vi "New_probe_ver6-rev_with_cycle.vi"() -> ()   [LabVIEW 2012]
panel:
  in  "Period [ms]":dbl=100.0
  in  "wait for stable [ms]":dbl=100.0
  in  "I for Lockin [A]":dbl
  out "X-Y":cluster{"X":dbl[], "Y":dbl[]}[](graph) caption="XY Graph"
  out "R 2":cluster{"X":dbl[], "Y":dbl[]}[](graph) caption="XY Graph"
  out "Lockin Y (V)":dbl=0.0511149801
  out "H":cluster{"X":dbl[], "Y":dbl[]}[](graph) caption="XY Graph"
  in  "X":string(combo)="100 uA"
  out "Lakeshore Reading (K)":dbl
  in  "Measure":bool
  in  "Y":string(combo)="100 uA"
  out "T":cluster{"X":dbl[], "Y":dbl[]}[](graph) caption="XY Graph"
  in  "Reset":bool
  out "R":cluster{"X":dbl[], "Y":dbl[]}[](graph) caption="XY Graph"
  in  "T:Lock in\nF:delta":bool
  out "Lockin X (V)":dbl=0.0511149801
  in  "Lockin SR830":refnum<visa-resource-name>="GPIB0::22::INSTR"
  in  "Keithley":refnum<visa-resource-name>="GPIB0::20::INSTR"
  in  "Arm Delta":bool
  in  "I-HIGH [A]":dbl=0.0001 format="%#_6e"
  in  "DELAY [sec]":dbl=0.002 format="%#_6e"
  in  "Compliance [V]":dbl=1.0 format="%#_6f"
  in  "Abort Delta":bool
  out "Delta Reading [Ohm]":dbl=0.0511149801
  in  "Input (0: A  1: B)":u16
  in  "Stop":bool
  in  "Lakeshore":refnum<visa-resource-name>="GPIB0::12::INSTR"
  in  "ramp [mT/sec]":dbl=3.0
  in  "step [ms]":dbl=100.0
  in  "set [mT]":dbl
  in  "Set field":bool
  in  "Initialize":bool
  out "Magnetic Field [mT]":dbl(knob) scale=-500.0..500.0
  in  "Save":bool
  in  "?":bool
  in  "error in (no error)":errorcluster
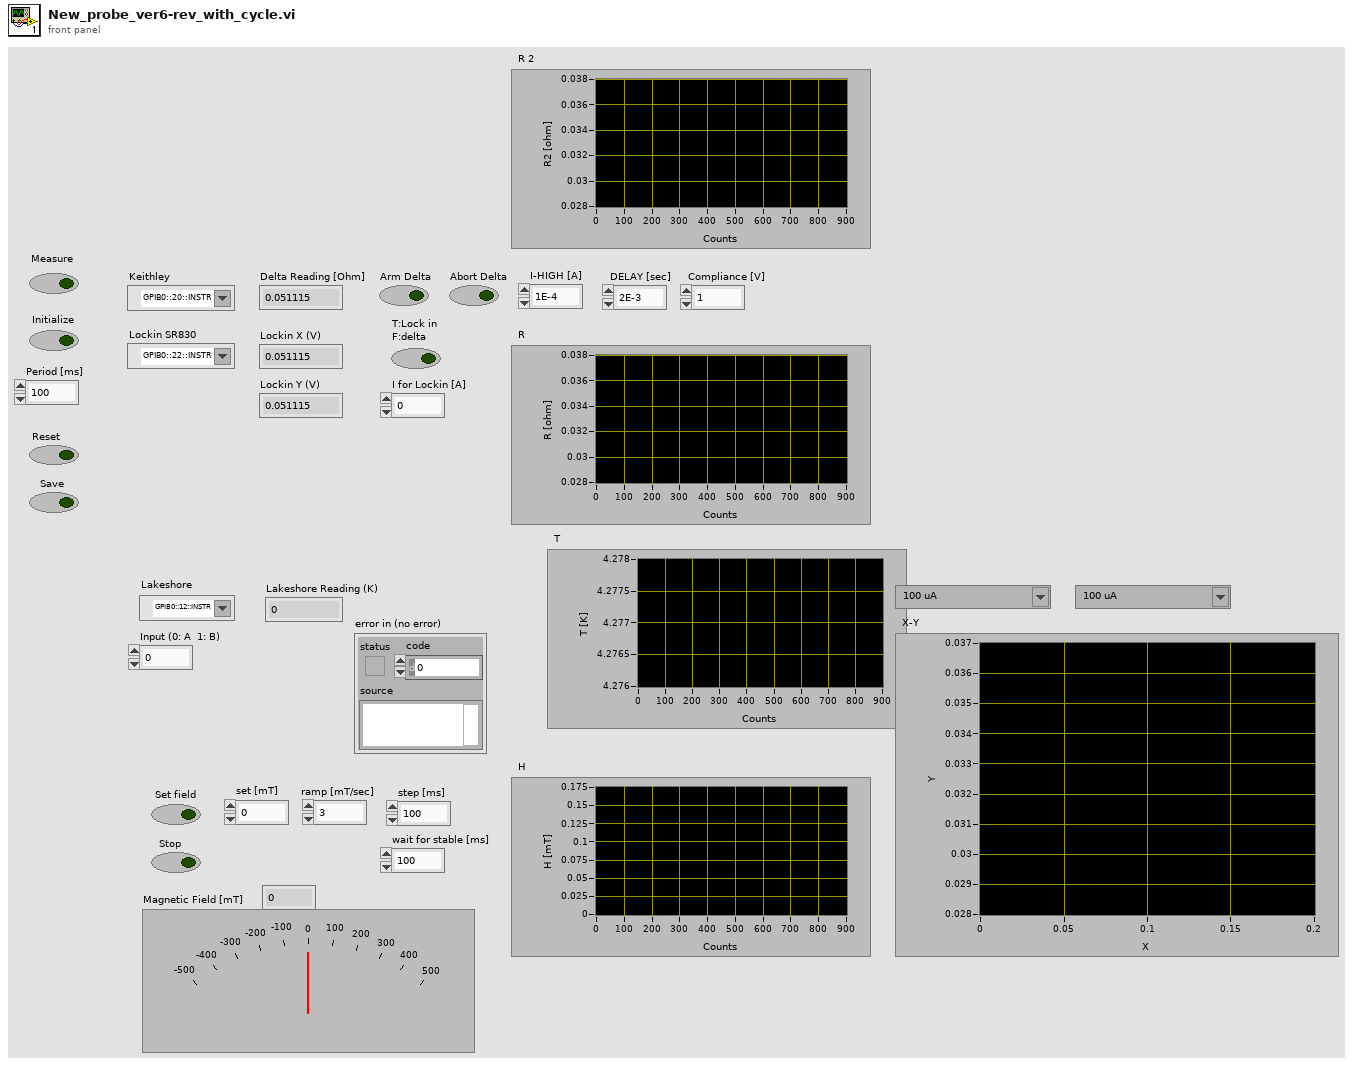
[diagram p1: front panel]
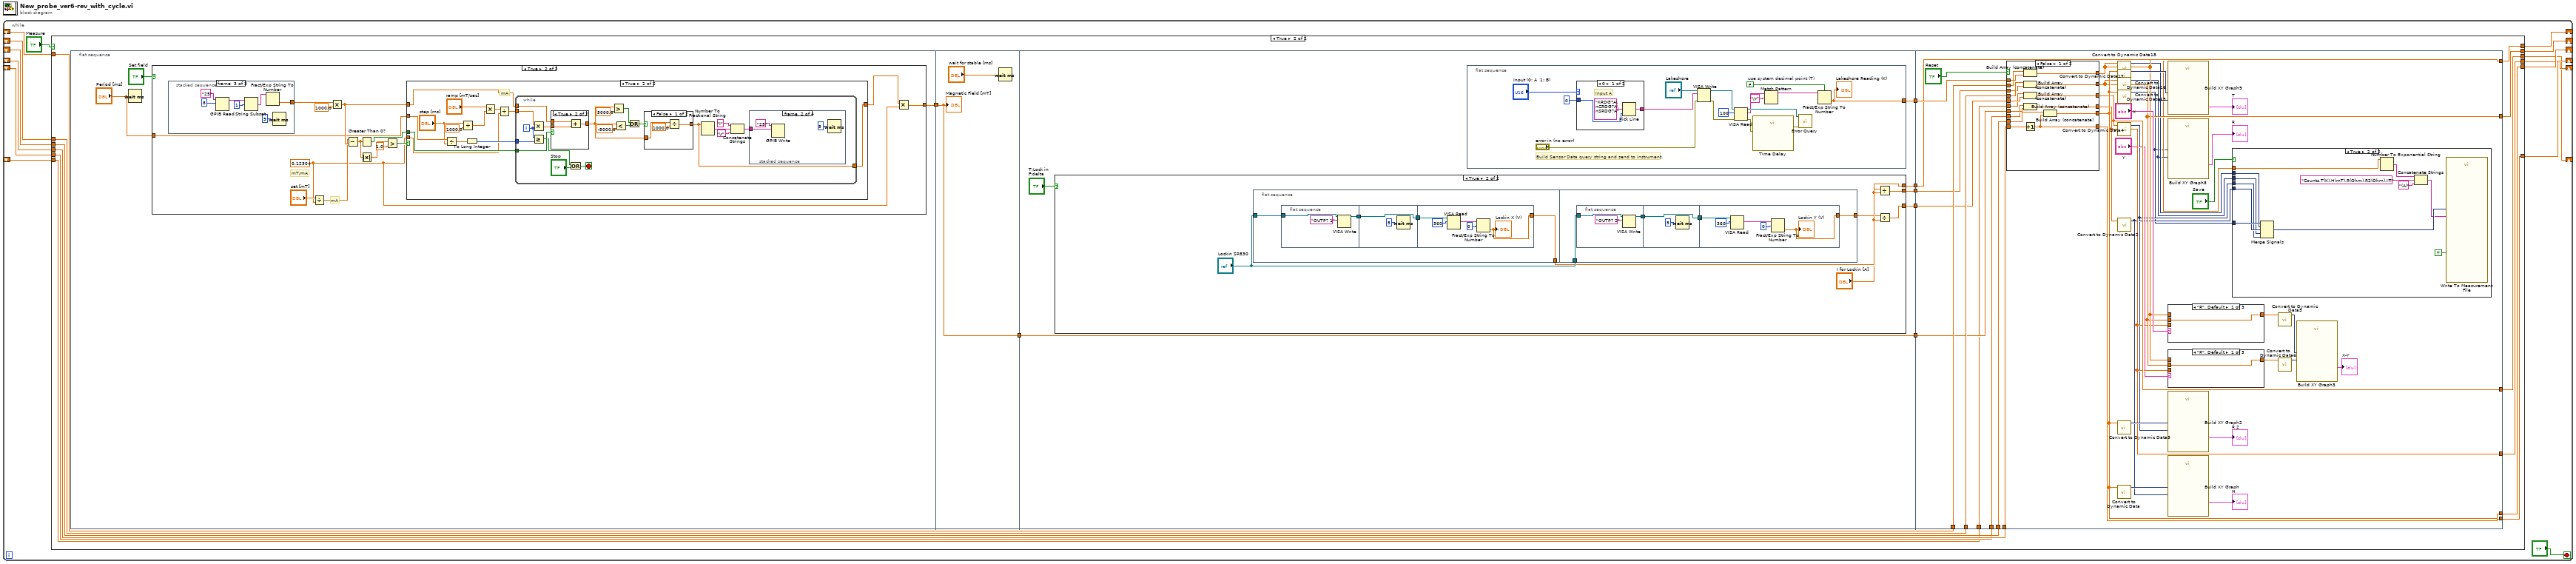
[diagram p0: block diagram]
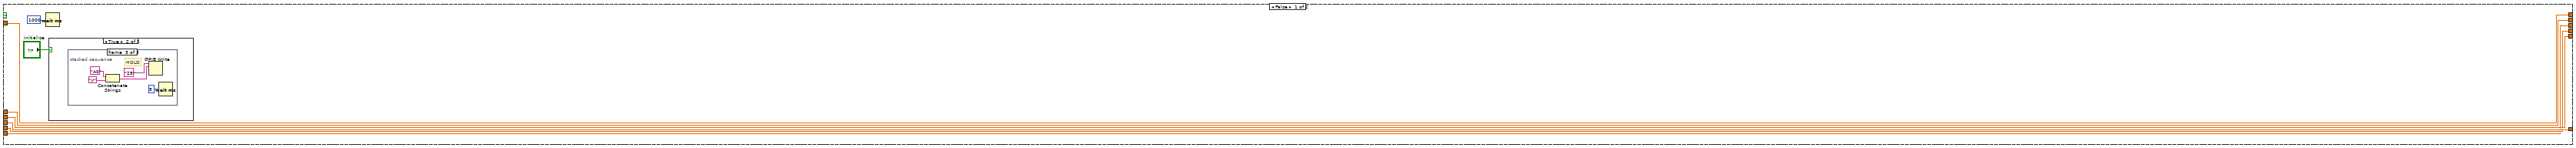
[diagram p2: hidden frame]
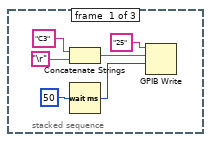
[diagram p4: hidden frame]
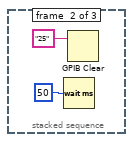
[diagram p5: hidden frame]
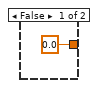
[diagram p6: hidden frame]
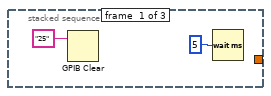
[diagram p7: hidden frame]
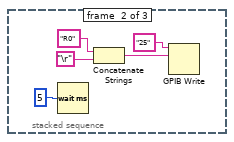
[diagram p8: hidden frame]
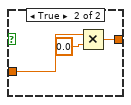
[diagram p10: hidden frame]
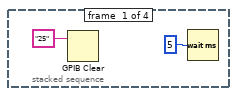
[diagram p11: hidden frame]
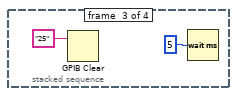
[diagram p12: hidden frame]
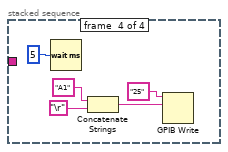
[diagram p13: hidden frame]
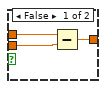
[diagram p14: hidden frame]
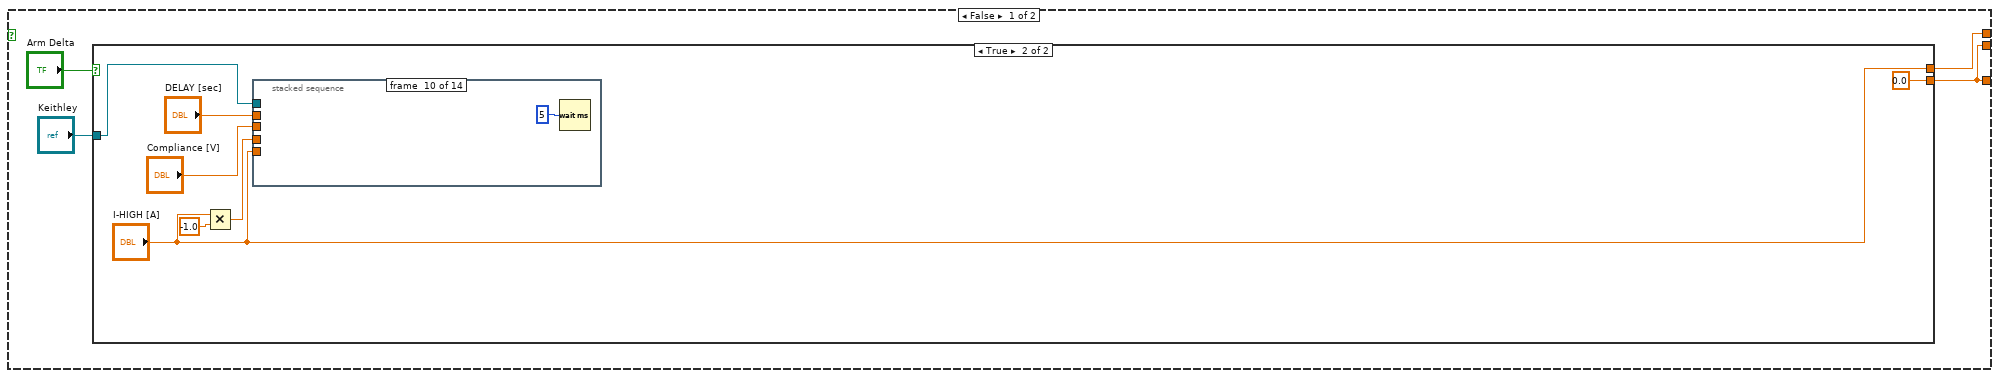
[diagram p15: hidden frame]
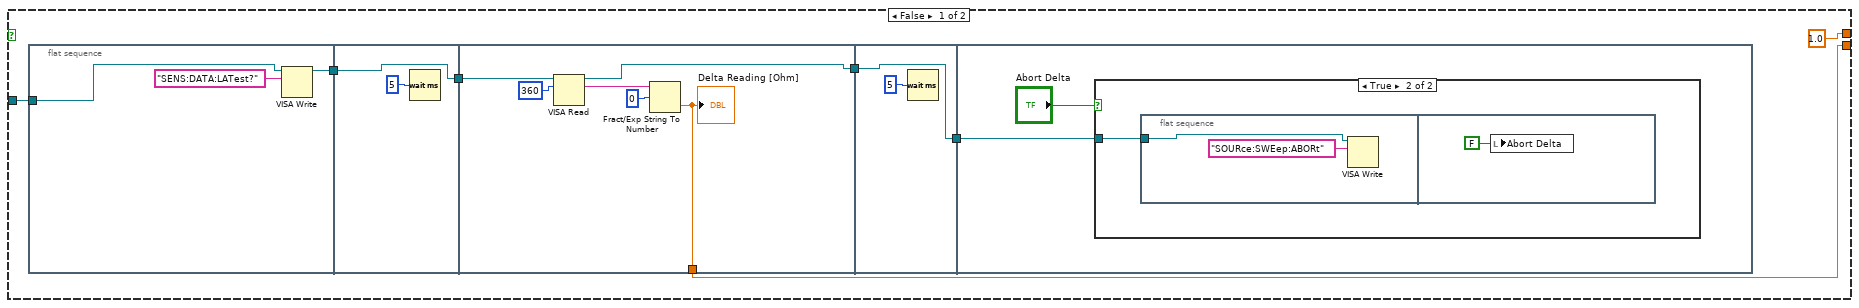
[diagram p16: hidden frame]
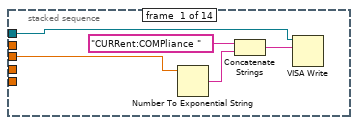
[diagram p18: hidden frame]
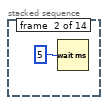
[diagram p19: hidden frame]
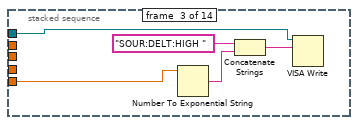
[diagram p20: hidden frame]
diagram:
  n1 = while {
    shift-right: [w13] -> _
    shift-left: _ -> [w6]
    shift-right: [w11] -> _
    shift-left: _ -> [w9]
    shift-right: [w10] -> _
    shift-left: _ -> [w8]
    shift-right: [w12] -> _
    shift-left: _ -> [w7]
    shift-right: [w4] -> _
    shift-left: _ -> [w3]
    shift-right: [w2] -> _
    shift-left: _ -> [w1]
    stop <- "?" stop-if-true
    n2 = case shown="True" "Measure" {
      tunnel: [w20 w51] -> w13
      tunnel: [w18 w50] -> w12
      tunnel: [w19 w49] -> w11
      tunnel: [w17 w48] -> w10
      tunnel: w9 -> [w19 w44]
      tunnel: w8 -> [w17 w45]
      tunnel: w7 -> [w18 w46]
      tunnel: w6 -> [w20 w47]
      tunnel: [w16 w41] -> w4
      tunnel: w3 -> [w16 w40]
      tunnel: [w15 w38] -> w2
      tunnel: w1 -> [w15 w37]
      frame False {
        n3 = Wait (ms)(milliseconds to wait=u32 1000) -> ()  [unwired: 1 out]
        n4 = case shown="True" "Initialize" {
          frame False {
          }
          frame True {
            n5 = stacked-sequence {
              frame #0 {
                n6 = Concatenate Strings("C3", "\r") -> (w24:string)
                n7 = Wait (ms)(milliseconds to wait=50) -> (millisecond timer value=w25:u32)
                n8 = GPIB Write(0:"25", 1:w24, 2:w25) -> ()  [unwired: 2 in, 2 out]
              }
              frame #1 {
                n9 = Wait (ms)(milliseconds to wait=50) -> ()  [unwired: 1 out]
                n10 = GPIB Clear(3:"25") -> ()  [unwired: 1 in, 2 out]
              }
              frame #2 {
                # "HOLD"
                n11 = Concatenate Strings("A0", "\r") -> (w32:string)
                n12 = GPIB Write(0:"25", 1:w32) -> ()  [unwired: 3 in, 2 out]
                n13 = Wait (ms)(milliseconds to wait=5) -> ()  [unwired: 1 out]
              }
            }
          }
        }
      }
      frame True {
        n14 = flat-sequence {
          tunnel: [w56] -> w54
          tunnel: w54 -> [w146]
          tunnel: [w146] -> w43
          tunnel: [w151] -> w53
          tunnel: [w150] -> w52
          tunnel: w43 -> [w149]
          tunnel: [w149] -> w42
          tunnel: [w148] -> w39
          tunnel: [w147] -> w36
          tunnel: [w312] -> w48
          tunnel: [w299] -> w50
          tunnel: [w290] -> w51
          tunnel: [w289] -> w49
          tunnel: w47 -> [w316]
          tunnel: w46 -> [w315]
          tunnel: w44 -> [w314]
          tunnel: w45 -> [w313]
          tunnel: w53 -> [w311]
          tunnel: w52 -> [w310]
          tunnel: w42 -> [w304]
          tunnel: w40 -> [w303]
          tunnel: [w288] -> w41
          tunnel: w39 -> [w302]
          tunnel: [w298] -> w38
          tunnel: w37 -> [w297]
          tunnel: w36 -> [w280]
          frame #0 {
            n15 = Wait (ms)(milliseconds to wait="Period [ms]") -> ()  [unwired: 1 out]
            n16 = case shown="True" "Set field" {
              tunnel: [0.0 w63] -> w56
              tunnel: "Period [ms]" -> [_ w62]
              frame False {
              }
              frame True {
                w59 = 0.12304
                # "mT/mA"
                # "mA"
                n17 = stacked-sequence {
                  tunnel: [_ _ w84] -> w67
                  frame #0 {
                    n18 = GPIB Clear(3:"25") -> ()  [unwired: 1 in, 2 out]
                    n19 = Wait (ms)(milliseconds to wait=5) -> ()  [unwired: 1 out]
                  }
                  frame #1 {
                    n20 = Wait (ms)(milliseconds to wait=5) -> ()  [unwired: 1 out]
                    n21 = Concatenate Strings("R0", "\r") -> (w76:string)
                    n22 = GPIB Write(0:"25", 1:w76) -> ()  [unwired: 3 in, 2 out]
                  }
                  frame #2 {
                    n23 = GPIB Read(0:"25", 1:8 ("count")) -> (5:w80:string)  [unwired: 3 in, 2 out]
                    n24 = String Subset(string=w80, offset (0)=1) -> (substring=w85:string)  [unwired: 1 in]
                    n25 = Fract/Exp String To Number(string=w85) -> (number=w84:dbl)  [unwired: 3 in, 1 out]
                    n26 = Wait (ms)(milliseconds to wait=5) -> ()  [unwired: 1 out]
                  }
                }
                n27 = Divide(x="set [mT]", y=w59) -> (x/y=w60:dbl)
                n28 = Multiply(x=w67, y=1000.0) -> (x*y=w66:dbl)
                n29 = Subtract(x=w60, y=w66) -> (x-y=w70:dbl)
                n30 = Greater Than 0?(x=w70) -> (x > 0?=w69:bool)
                n31 = Absolute Value(x=w70) -> (abs(x)=w71:dbl)
                n32 = Greater?(x=w71, y=1.0) -> (0:w65:bool)
                n33 = case shown="True" w65 {
                  tunnel: w66 -> [w87 w100]
                  tunnel: w69 -> [_ w99]
                  tunnel: [w87 w98] -> w64
                  tunnel: w62 -> [_ w95]
                  tunnel: w59 -> [_ w89]
                  frame False {
                  }
                  frame True {
                    # "mA"
                    n34 = Divide(x=w95, y="step [ms]") -> (x/y=w96:dbl)
                    n35 = Divide(x="step [ms]", y=1000.0) -> (x/y=w94:dbl)
                    n36 = To Long Integer(number=w96) -> (32bit integer=w97:i32)
                    n37 = Multiply(x="ramp [mT/sec]", y=w94) -> (x*y=w90:dbl)
                    n38 = Divide(x=w90, y=w89) -> (x/y=w88:dbl)
                    n39 = while {
                      tunnel: w100 -> [w118]
                      tunnel: w88 -> [w117]
                      tunnel: w99 -> [w114]
                      tunnel: w97 -> [w105]
                      tunnel: [w101] -> w98
                      i -> [w106]
                      stop <- w103 stop-if-true
                      n40 = Multiply(x=w117, y=w106) -> (x*y=w116:dbl)
                      n41 = Greater Or Equal?(x=w106, y=w105) -> (x >= y?=w104:bool)
                      n42 = case shown="True" w114 {
                        tunnel: w118 -> [w140 w144]
                        tunnel: w116 -> [w141 w143]
                        tunnel: [w139 w142] -> w108
                        frame False {
                          n43 = Subtract(x=w140, y=w141) -> (x-y=w139:dbl)
                        }
                        frame True {
                          n44 = Add(x=w144, y=w143) -> (x+y=w142:dbl)
                        }
                      }
                      n45 = Or(x=w104, y="Stop") -> (x .or. y?=w103:bool)
                      n46 = Greater?(x=w108, y=5000.0) -> (0:w110:bool)
                      n47 = Less?(x=w108, y=-5000.0) -> (x < y?=w109:bool)
                      n48 = Or(x=w110, y=w109) -> (x .or. y?=w107:bool)
                      n49 = case shown="False" w107 {
                        tunnel: [w121 w126] -> w101
                        tunnel: w108 -> [w122 w125]
                        frame False {
                          n50 = Divide(x=w122, y=1000.0) -> (x/y=w121:dbl)
                        }
                        frame True {
                          n51 = Multiply(x=w125, y=0.0) -> (x*y=w126:dbl)
                        }
                      }
                      n52 = Number To Fractional String(number=w101) -> (F-format string=w115:string)  [unwired: 3 in]
                      n53 = Concatenate Strings("I", w115, "\r") -> (w119:string)
                      n54 = stacked-sequence {
                        tunnel: w119 -> [_ w130 _ _]
                        frame #0 {
                          n55 = GPIB Clear(3:"25") -> ()  [unwired: 1 in, 2 out]
                          n56 = Wait (ms)(milliseconds to wait=5) -> ()  [unwired: 1 out]
                        }
                        frame #1 {
                          n57 = GPIB Write(0:"25", 1:w130) -> ()  [unwired: 3 in, 2 out]
                          n58 = Wait (ms)(milliseconds to wait=5) -> ()  [unwired: 1 out]
                        }
                        frame #2 {
                          n59 = GPIB Clear(3:"25") -> ()  [unwired: 1 in, 2 out]
                          n60 = Wait (ms)(milliseconds to wait=5) -> ()  [unwired: 1 out]
                        }
                        frame #3 {
                          n61 = Wait (ms)(milliseconds to wait=5) -> ()  [unwired: 1 out]
                          n62 = Concatenate Strings("A1", "\r") -> (w135:string)
                          n63 = GPIB Write(0:"25", 1:w135) -> ()  [unwired: 3 in, 2 out]
                        }
                      }
                    }
                  }
                }
                n64 = Multiply(x=w64, y=w59) -> (x*y=w63:dbl)
              }
            }
          }
          frame #1 {
            n65 = Wait (ms)(milliseconds to wait="wait for stable [ms]") -> ()  [unwired: 1 out]
            "Magnetic Field [mT]" <- w146
          }
          frame #2 {
            n66 = case shown="True" "T:Lock in\nF:delta" {
              tunnel: [w154 w226] -> w150
              tunnel: [w154 w224] -> w148
              tunnel: [w153 "I for Lockin [A]"] -> w147
              frame False {
                n67 = case shown="True" "Arm Delta" {
                  tunnel: [w159 0.0] -> w154
                  tunnel: "Keithley" -> [w158 w184]
                  tunnel: [1.0 ("I-HIGH [A]") "I-HIGH [A]"] -> w153
                  frame False {
                    n68 = flat-sequence {
                      tunnel: [w165] -> w162
                      tunnel: w158 -> [w164]
                      tunnel: [w167] -> w163
                      tunnel: w162 -> [w167]
                      tunnel: w163 -> [w171]
                      tunnel: [w170] -> w160
                      tunnel: [w169] -> w159
                      tunnel: [w175] -> w161
                      tunnel: w160 -> [w175]
                      tunnel: w161 -> [w177]
                      frame #0 {
                        n69 = VISA Write(VISA resource name=w164, write buffer="SENS:DATA:LATest?" ("write buffer 2")) -> (VISA resource name out=w165:refnum<visa-resource-name>)  [unwired: 1 in, 2 out]
                      }
                      frame #1 {
                        n70 = Wait (ms)(milliseconds to wait=5) -> ()  [unwired: 1 out]
                      }
                      frame #2 {
                        n71 = VISA Read(VISA resource name=w171, byte count=u32 360) -> (VISA resource name out=w170:refnum<visa-resource-name>, read buffer=w173:string)  [unwired: 1 in, 2 out]
                        n72 = Fract/Exp String To Number(string=w173, offset=0) -> (number=w169:dbl)  [unwired: 3 out]
                        "Delta Reading [Ohm]" <- w169
                      }
                      frame #3 {
                        n73 = Wait (ms)(milliseconds to wait=5) -> ()  [unwired: 1 out]
                      }
                      frame #4 {
                        n74 = case shown="True" "Abort Delta" {
                          tunnel: w177 -> [_ w179]
                          frame False {
                          }
                          frame True {
                            n75 = flat-sequence {
                              tunnel: w179 -> [w181]
                              frame #0 {
                                n76 = VISA Write(VISA resource name=w181, write buffer="SOURce:SWEep:ABORt") -> ()  [unwired: 1 in, 3 out]
                              }
                              frame #1 {
                                n77 = local write "Abort Delta"(FALSE) -> ()
                              }
                            }
                          }
                        }
                      }
                    }
                  }
                  frame True {
                    n78 = Multiply(x="I-HIGH [A]", y=-1.0) -> (x*y=w188:dbl)
                    n79 = stacked-sequence {
                      tunnel: "I-HIGH [A]" -> [_ _ w198 _ _ _ _ _ _ _ _ _ _ _]
                      tunnel: w184 -> [w191 _ w196 _ w203 _ w209 _ w214 _ w217 _ w220 _]
                      tunnel: w188 -> [_ _ _ _ w202 _ _ _ _ _ _ _ _ _]
                      tunnel: "DELAY [sec]" -> [_ _ _ _ _ _ w208 _ _ _ _ _ _ _]
                      tunnel: "Compliance [V]" -> [w190 _ _ _ _ _ _ _ _ _ _ _ _ _]
                      frame #0 {
                        n80 = Number To Exponential String(number=w190) -> (E-format string=w193:string)  [unwired: 3 in]
                        n81 = Concatenate Strings("CURRent:COMPliance ", w193) -> (w192:string)
                        n82 = VISA Write(VISA resource name=w191, write buffer=w192) -> ()  [unwired: 1 in, 3 out]
                      }
                      frame #1 {
                        n83 = Wait (ms)(milliseconds to wait=5) -> ()  [unwired: 1 out]
                      }
                      frame #2 {
                        n84 = Number To Exponential String(number=w198) -> (E-format string=w199:string)  [unwired: 3 in]
                        n85 = Concatenate Strings("SOUR:DELT:HIGH ", w199) -> (w197:string)
                        n86 = VISA Write(VISA resource name=w196, write buffer=w197) -> ()  [unwired: 1 in, 3 out]
                      }
                      frame #3 {
                        n87 = Wait (ms)(milliseconds to wait=5) -> ()  [unwired: 1 out]
                      }
                      frame #4 {
                        n88 = Number To Exponential String(number=w202) -> (E-format string=w205:string)  [unwired: 3 in]
                        n89 = Concatenate Strings("SOUR:DELT:LOW ", w205) -> (w204:string)
                        n90 = VISA Write(VISA resource name=w203, write buffer=w204) -> ()  [unwired: 1 in, 3 out]
                      }
                      frame #5 {
                        n91 = Wait (ms)(milliseconds to wait=5) -> ()  [unwired: 1 out]
                      }
                      frame #6 {
                        n92 = Number To Exponential String(number=w208) -> (E-format string=w211:string)  [unwired: 3 in]
                        n93 = Concatenate Strings("SOUR:DELT:DELay ", w211) -> (w210:string)
                        n94 = VISA Write(VISA resource name=w209, write buffer=w210) -> ()  [unwired: 1 in, 3 out]
                      }
                      frame #7 {
                        n95 = Wait (ms)(milliseconds to wait=5) -> ()  [unwired: 1 out]
                      }
                      frame #8 {
                        n96 = VISA Write(VISA resource name=w214, write buffer="UNIT OHMS ") -> ()  [unwired: 1 in, 3 out]
                      }
                      frame #9 {
                        n97 = Wait (ms)(milliseconds to wait=5) -> ()  [unwired: 1 out]
                      }
                      frame #10 {
                        n98 = VISA Write(VISA resource name=w217, write buffer="DELTa:ARM") -> ()  [unwired: 1 in, 3 out]
                      }
                      frame #11 {
                        n99 = Wait (ms)(milliseconds to wait=3000) -> ()  [unwired: 1 out]
                      }
                      frame #12 {
                        n100 = VISA Write(VISA resource name=w220, write buffer="INIT:IMM") -> ()  [unwired: 1 in, 3 out]
                      }
                      frame #13 {
                        n101 = local write "Arm Delta"(FALSE) -> ()
                      }
                    }
                  }
                }
              }
              frame True {
                n102 = flat-sequence {
                  tunnel: [w230] -> w227
                  tunnel: "Lockin SR830" -> [w229]
                  tunnel: "Lockin SR830" -> [w244]
                  tunnel: [w243] -> w225
                  frame #0 {
                    n103 = flat-sequence {
                      tunnel: w229 -> [w235]
                      tunnel: [w233] -> w232
                      tunnel: [w236] -> w231
                      tunnel: w232 -> [w236]
                      tunnel: w231 -> [w240]
                      tunnel: [w238] -> w230
                      frame #0 {
                        n104 = VISA Write(VISA resource name=w235, write buffer="OUTP? 1" ("write buffer 2")) -> (VISA resource name out=w233:refnum<visa-resource-name>)  [unwired: 1 in, 2 out]
                      }
                      frame #1 {
                        n105 = Wait (ms)(milliseconds to wait=5) -> ()  [unwired: 1 out]
                      }
                      frame #2 {
                        n106 = VISA Read(VISA resource name=w240, byte count=u32 360) -> (read buffer=w239:string)  [unwired: 1 in, 3 out]
                        n107 = Fract/Exp String To Number(string=w239, offset=0) -> (number=w238:dbl)  [unwired: 3 out]
                        "Lockin X (V)" <- w238
                      }
                    }
                  }
                  frame #1 {
                    n108 = flat-sequence {
                      tunnel: w244 -> [w249]
                      tunnel: [w247] -> w246
                      tunnel: [w250] -> w245
                      tunnel: w246 -> [w250]
                      tunnel: w245 -> [w254]
                      tunnel: [w252] -> w243
                      frame #0 {
                        n109 = VISA Write(VISA resource name=w249, write buffer="OUTP? 2" ("write buffer 2")) -> (VISA resource name out=w247:refnum<visa-resource-name>)  [unwired: 1 in, 2 out]
                      }
                      frame #1 {
                        n110 = Wait (ms)(milliseconds to wait=5) -> ()  [unwired: 1 out]
                      }
                      frame #2 {
                        n111 = VISA Read(VISA resource name=w254, byte count=u32 360) -> (read buffer=w253:string)  [unwired: 1 in, 3 out]
                        n112 = Fract/Exp String To Number(string=w253, offset=0) -> (number=w252:dbl)  [unwired: 3 out]
                        "Lockin Y (V)" <- w252
                      }
                    }
                  }
                }
                n113 = Divide(x=w227, y="I for Lockin [A]") -> (x/y=w226:dbl)
                n114 = Divide(x=w225, y="I for Lockin [A]") -> (x/y=w224:dbl)
              }
            }
            n115 = flat-sequence {
              tunnel: [w257] -> w151
              frame #0 {
                w265 = FALSE  # use system decimal point (T)
                # "Build Sensor Data query string and send to instrument."
                n116 = case shown="0" "Input (0: A  1: B)" {
                  tunnel: u16 0 ("Input (0: A)") -> [w274 w276]
                  tunnel: [w273 w277] -> w263
                  frame 0 {
                    # "Input A"
                    n117 = Pick Line(multi-line string="KRDG?A\nCRDG?A\nSRDG?A", line index=w274) -> (output string=w273:string)  [unwired: 1 in]
                  }
                  frame 1, Default {
                    # "Input B"
                    n118 = Pick Line(multi-line string="KRDG?B\nCRDG?B\nSRDG?B", line index=w276) -> (output string=w277:string)  [unwired: 1 in]
                  }
                }
                n119 = VISA Write(VISA resource name="Lakeshore", write buffer=w263, error in (no error)="error in (no error)") -> (VISA resource name out=w267:refnum<visa-resource-name>, error out=w266:errorcluster)  [unwired: 1 out]
                n120 = VISA Read(VISA resource name=w267, byte count=100, error in (no error)=w266) -> (VISA resource name out=w271:refnum<visa-resource-name>, read buffer=w269:string, error out=w261:errorcluster)  [unwired: 1 out]
                n121 = call "Time Delay"("error in (no error)"=w261) -> ("error out"=w262:errorcluster)  [unwired: 10 in]
                n122 = Match Pattern(string=w269, regular expression="\\r") -> (before substring=w264:string)  [unwired: 1 in, 3 out]
                n123 = call "Error Query.vi"("error in (no error)"=w262, "VISA resource name"=w271) -> ()  [unwired: 7 in, 3 out]
                n124 = Fract/Exp String To Number(use system decimal point (T)=w265, string=w264) -> (number=w257:dbl)  [unwired: 2 in, 1 out]
                "Lakeshore Reading (K)" <- w257
              }
            }
          }
          frame #3 {
            n125 = case shown="False" "Reset" {
              tunnel: w311 -> [w346 _]
              tunnel: [w350 dbl[] []] -> w290
              tunnel: [w349 dbl[] []] -> w289
              tunnel: w314 -> [w348 _]
              tunnel: w310 -> [w347 _]
              tunnel: w316 -> [w345 _]
              tunnel: [w344 dbl[] []] -> w299
              tunnel: w315 -> [w343 _]
              tunnel: w313 -> [w342 _]
              tunnel: [w341 0.0] -> w312
              tunnel: w304 -> [w340 _]
              tunnel: [w339 dbl[] []] -> w288
              tunnel: w303 -> [w338 _]
              tunnel: [w337 dbl[] []] -> w298
              tunnel: w302 -> [w336 _]
              tunnel: w297 -> [w335 _]
              frame False {
                n126 = Build Array (concatenate)(w345, w346) -> (w350:dbl[])
                n127 = Build Array (concatenate)(w348, w347) -> (w349:dbl[])
                n128 = Build Array (concatenate)(w335, w336) -> (w337:dbl[])
                n129 = Build Array (concatenate)(w338, w340) -> (w339:dbl[])
                n130 = Increment(x=w342) -> (x+1=w341:dbl)
                n131 = Build Array (concatenate)(w343, w341) -> (w344:dbl[])
              }
              frame True {
                n132 = local write "Reset"(FALSE) -> ()
              }
            }
            n133 = call "Convert to Dynamic Data17"("Array"=w299) -> ("Dynamic Data Type"=w307:dynamicdata)  [unwired: 3 in]
            n134 = call "Convert to Dynamic Data3"("Array"=w299) -> ("Dynamic Data Type"=w300:dynamicdata)  [unwired: 3 in]
            n135 = call "Convert to Dynamic Data"("Array"=w299) -> ("Dynamic Data Type"=w285:dynamicdata)  [unwired: 3 in]
            n136 = call "Convert to Dynamic Data18"("Array"=w290) -> ("Dynamic Data Type"=w284:dynamicdata)  [unwired: 3 in]
            n137 = call "Convert to Dynamic Data16"("Array"=w289) -> ("Dynamic Data Type"=w282:dynamicdata)  [unwired: 3 in]
            n138 = call "Convert to Dynamic Data15"("Array"=w299) -> ("Dynamic Data Type"=w279:dynamicdata)  [unwired: 3 in]
            n139 = call "Convert to Dynamic Data4"("Array"=w298) -> ("Dynamic Data Type"=w281:dynamicdata)  [unwired: 3 in]
            n140 = call "Convert to Dynamic Data2"("Array"=w288) -> ("Dynamic Data Type"=w283:dynamicdata)  [unwired: 3 in]
            n141 = call "Build XY Graph9"("Y Input"=w284, "X Input"=w307) -> ("XY Graph"=→"T":cluster{"X":dbl[], "Y":dbl[]}[])  [unwired: 8 in, 1 out]
            n142 = call "Build XY Graph8"("Y Input"=w282, "X Input"=w279) -> ("XY Graph"=→"R":cluster{"X":dbl[], "Y":dbl[]}[])  [unwired: 8 in, 1 out]
            n143 = case shown="\"R\", Default" "X" {
              tunnel: [w332 w333 w334] -> w292
              tunnel: w289 -> [w332 _ _]
              tunnel: w290 -> [_ w333 _]
              tunnel: w288 -> [_ _ w334]
              frame "R", Default {
              }
              frame "T" {
              }
              frame "H" {
              }
            }
            n144 = case shown="\"R\", Default" "Y" {
              tunnel: [w329 w330 w331] -> w291
              tunnel: w289 -> [w329 _ _]
              tunnel: w290 -> [_ w330 _]
              tunnel: w288 -> [_ _ w331]
              frame "R", Default {
              }
              frame "T" {
              }
              frame "H" {
              }
            }
            n145 = call "Build XY Graph2"("Y Input"=w281, "X Input"=w300) -> ("XY Graph"=→"R 2":cluster{"X":dbl[], "Y":dbl[]}[])  [unwired: 8 in, 1 out]
            n146 = call "Build XY Graph"("Y Input"=w283, "X Input"=w285) -> ("XY Graph"=→"H":cluster{"X":dbl[], "Y":dbl[]}[])  [unwired: 8 in, 1 out]
            n147 = case shown="True" "Save" {
              tunnel: w279 -> [_ w326]
              tunnel: w284 -> [_ w325]
              tunnel: w283 -> [_ w324]
              tunnel: w282 -> [_ w323]
              tunnel: w281 -> [_ w322]
              tunnel: w280 -> [_ w321]
              frame False {
              }
              frame True {
                n148 = Merge Signals(w326, w325, w324, w323, w322) -> (w327:dynamicdata)
                n149 = Number To Exponential String(number=w321) -> (E-format string=w319:string)  [unwired: 3 in]
                n150 = Concatenate Strings(w319, "Counts,T(K),H(mT),R(Ohm),R2(Ohm),I=", "(A)") -> (w318:string)
                n151 = call "Write To Measurement File"("Signals"=w327, "Reset"=TRUE, "Comment"=w318) -> ()  [unwired: 14 in, 3 out]
              }
            }
            n152 = call "Convert to Dynamic Data5"("Array"=w292) -> ("Dynamic Data Type"=w294:dynamicdata)  [unwired: 3 in]
            n153 = call "Convert to Dynamic Data6"("Array"=w291) -> ("Dynamic Data Type"=w295:dynamicdata)  [unwired: 3 in]
            n154 = call "Build XY Graph3"("Y Input"=w295, "X Input"=w294) -> ("XY Graph"=→"X-Y":cluster{"X":dbl[], "Y":dbl[]}[])  [unwired: 8 in, 1 out]
          }
        }
      }
    }
  }
